vi "81_Ultrasonic Example.vi"() -> ()   [LabVIEW 2018]
uses:
  <userlib>/KNR OS 3.0 LabVIEW Toolkit/Type Definition/Resource.ctl
  <userlib>/KNR OS 3.0 LabVIEW Toolkit/Type Definition/Ultrasonic Port Number.ctl
panel:
  in  "IP":string(combo)="172.22.11.2"
  in  "Port (US1-US4 for KNR)":T1 items=["US1-US4"=0, "US5-US8"=2]
  in  "Resource":T2=enum."KNRm_DDDD"
  out "Ultrasonic output":T3
  in  "Trigger Width (uS)":u32=5
  in  "Pulse Period (uS)":u32=10000
  in  "stop":bool
  # "KNRm does not require to\nconnect the terminal \"Port\". \nIt outputs a cluster : \nDist1(cm)=US1\nDist2(cm)=US2"
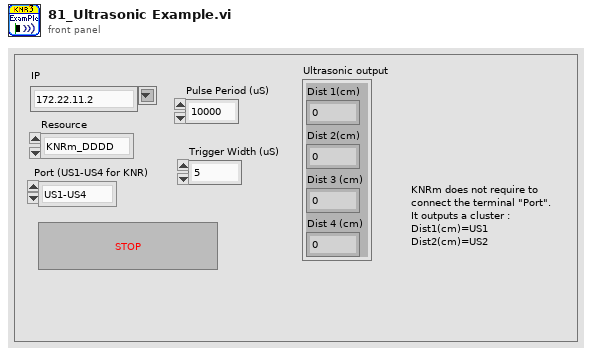
[diagram p1: front panel]
types:
  T1 = typedef "Ultrasonic Port Number.ctl" = u16
  T2 = typedef "Resource.ctl" = enum16{"KNRm_DDRC", "KNRm_DDDD", "KNRm_DDDR", "KNRm_DDDC", "KNR"}
  T3 = cluster{"Dist 1(cm)":dbl, "Dist 2(cm)":dbl, "Dist 3 (cm)":dbl, "Dist 4 (cm)":dbl}
  T4 = typedef "KNR3 Reference.ctl" = cluster{"FPGA Session":refnum<class "FPGA Interface Base.lvclass">, "Resource":T2}
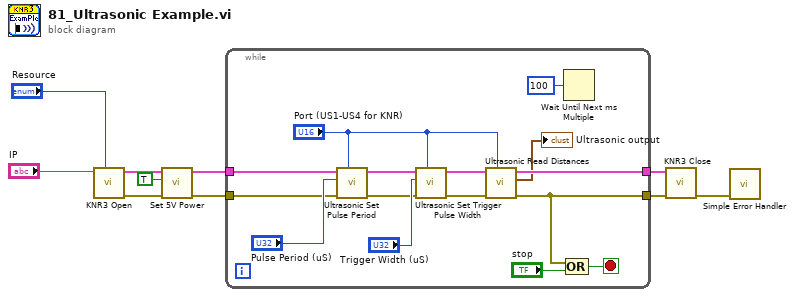
[diagram p0: block diagram]
diagram:
  n1 = call <userlib>:"KNR3 Open.vi"("Resource"="Resource", "IP"="IP") -> ("error out"=w5:errorcluster, "KNR out"=w10:T4)  [unwired: 8 in]
  n2 = call <userlib>:"Set 5V Power.vi"("error in (no error)"=w5, "5V Power(T)"=TRUE ("5V Power"), "KNR in"=w10) -> ("error out"=w4:errorcluster, "KNR out"=w6:T4)  [unwired: 7 in]
  n3 = while {
    tunnel: w6 -> [w25]
    tunnel: [w22] -> w9
    tunnel: w4 -> [w19]
    tunnel: [w14] -> w8
    stop <- w15 stop-if-true
    n4 = call <userlib>:"Ultrasonic Set Pulse Period.vi"("Port (US1-US4 for KNR)"="Port (US1-US4 for KNR)", "error in (no error)"=w19, "Pulse Period (10000 uS)"="Pulse Period (uS)", "KNR in"=w25) -> ("error out"=w18:errorcluster, "KNR out"=w24:T4)  [unwired: 6 in]
    n5 = call <userlib>:"Ultrasonic Set Trigger Pulse Width.vi"("Port (US1-US4 for KNR)"="Port (US1-US4 for KNR)", "error in (no error)"=w18, "Trigger Width (5 uS)"="Trigger Width (uS)", "KNR in"=w24) -> ("error out"=w17:errorcluster, "KNR out"=w23:T4)  [unwired: 6 in]
    n6 = call <userlib>:"Ultrasonic Read Distances.vi"("Port (US1-US4 for KNR)"="Port (US1-US4 for KNR)", "error in (no error)"=w17, "KNR in"=w23) -> ("error out"=w14:errorcluster, "Ultrasonic output"=→"Ultrasonic output":T3, "KNR out"=w22:T4)  [unwired: 6 in]
    n7 = Wait Until Next ms Multiple(millisecond multiple=u32 100) -> ()  [unwired: 1 out]
    n8 = Compound Arithmetic op=OR(w14, "stop") -> (w15:bool)
  }
  n9 = call <userlib>:"KNR3 Close.vi"("error in (no error)"=w8, "KNR in"=w9) -> ("error out"=w7:errorcluster)  [unwired: 9 in]
  n10 = call <vilib>:"Simple Error Handler.vi"("error in (no error)"=w7) -> ()  [unwired: 4 in, 5 out]
